vi "Valid.vi"(11 "BooleanPanel in":refnum<class "BooleanPanel.lvclass">) -> (2 "Issues":string[](array[string]))   [LabVIEW 2020]
uses:
  BooleanPanel.lvclass
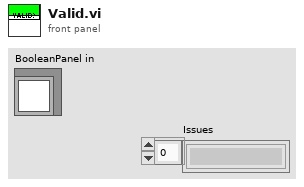
[diagram p1: front panel]
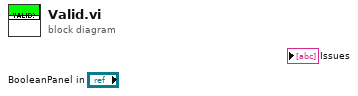
[diagram p0: block diagram]
diagram:
